vi "Read UI Object.vi"(8 "error in (no error)":errorcluster, 11 "Flex UI (Actor) in":refnum<class "Flex UI (Actor).lvclass">) -> (0 "error out":errorcluster, 2 "Flex UI Object":refnum<class "Flex UI.lvclass">, 3 "Flex UI (Actor) out":refnum<class "Flex UI (Actor).lvclass">)   [LabVIEW 2016, in "Flex UI (Parent Actor).lvlib" / "Flex UI (Actor).lvclass"]
uses:
  Flex UI (Actor).lvclass
  <vilib>/East West Architects/Flex UI/Flex UI (Parent)/Flex UI.lvclass
  Flex UI (Actor).lvclass/Flex UI (Actor).ctl
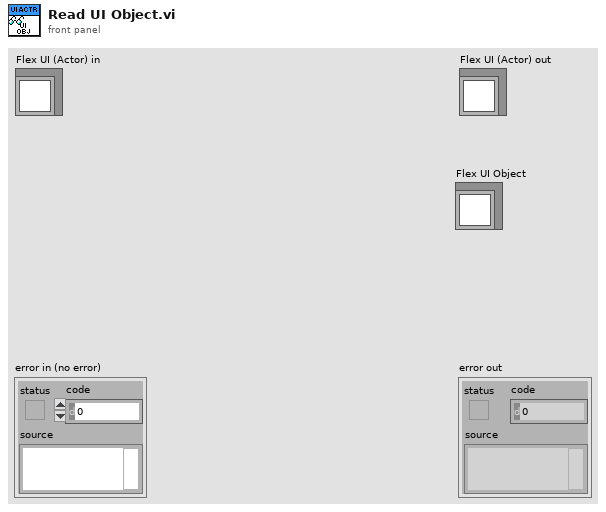
[diagram p1: front panel]
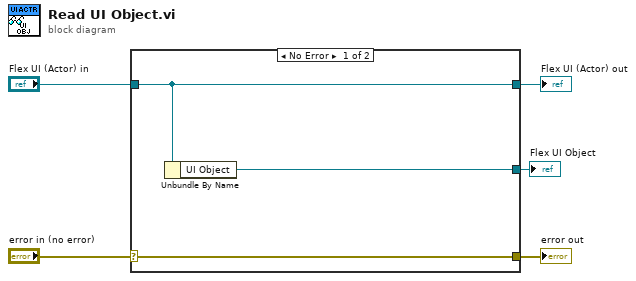
[diagram p0: block diagram]
diagram:
  n1 = case shown="No Error" "error in (no error)" {
    selector: "error in (no error)" -> [w8 w9]
    tunnel: [w8 w9] -> w4
    tunnel: [w7 w10] -> w2
    tunnel: "Flex UI (Actor) in" -> [w7 w10]
    tunnel: [w6 _] -> w1
    frame No Error {
      n2 = Unbundle By Name(w7) -> ("UI Object"=w6:refnum<class "Flex UI.lvclass">)
    }
    frame Error {
    }
  }
  "error out" <- w4
  "Flex UI (Actor) out" <- w2
  "Flex UI Object" <- w1
